vi "LI-U8 convert U8 array number to U32.vi"(4 "Large number -U8":T1) -> (1 "U32":u32, 2 "Roll-over?":bool)   [LabVIEW 2012]
doc: "Converts a large integer in U8 array format to U32, if it is not possible without rollover the boolean \"rollover?\" =T."
uses:
  User Access Type defs/Large number - U8 array.ctl
panel:
  # "<<LSD"
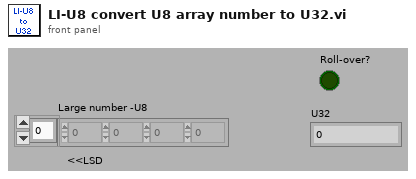
[diagram p1: front panel]
types:
  T1 = typedef "Large number - U8 array.ctl" = u8[]
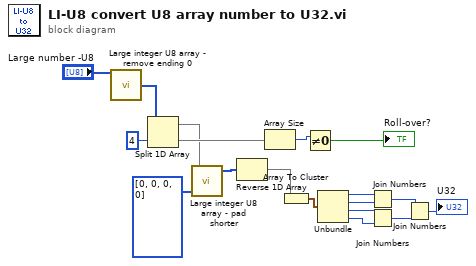
[diagram p0: block diagram]
diagram:
  n1 = call "Large integer U8 array - remove ending 0.vi"("Large number - U8"="Large number -U8") -> ("MSD zeros removed"=w16:T1)  [unwired: 4 out]
  n2 = Split 1D Array(array=w16, index=4) -> (first subarray=w2:T1, second subarray=w6:T1)
  n3 = call "Large integer U8 array - pad shorter.vi"("Large number -U8 2"=T1 [0, 0, 0, 0], "Large number -U8 1"=w2) -> ("Large number -U8 1 out"=w3:T1)  [unwired: 3 out]
  n4 = Reverse 1D Array(array=w3) -> (reversed array=w14:T1)
  n5 = Array Size(array=w6) -> (size(s)=w5:i32)
  n6 = Array To Cluster(array=w14) -> (cluster=w17:cluster{"[0]":u8, "[1]":u8, "[2]":u8, "[3]":u8})
  n7 = Not Equal To 0?(x=w5) -> (x != 0?=→"Roll-over?":bool)
  n8 = Unbundle(w17) -> ("[0]"=w13:u8, "[1]"=w12:u8, "[2]"=w11:u8, "[3]"=w10:u8)
  n9 = Join Numbers(hi=w13, lo=w12) -> ((hi.lo)=w8:u16)
  n10 = Join Numbers(hi=w11, lo=w10) -> ((hi.lo)=w7:u16)
  n11 = Join Numbers(hi=w8, lo=w7) -> ((hi.lo)=→"U32":u32)
